vi "StopSplashScreen.vi"(8 "error in (no error)":errorcluster) -> (0 "error out":errorcluster)   [LabVIEW 2011]
uses:
  EnumFgvEventCommand.ctl
  ToSplashScreen.ctl
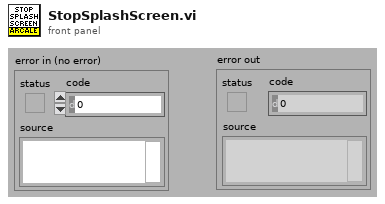
[diagram p1: front panel]
types:
  T1 = typedef "ToSplashScreen.ctl" = cluster{"Command":enum16{"Stop"}}
  T2 = typedef "EnumFgvEventCommand.ctl" = enum16{"Setup", "Cleanup", "Get"}
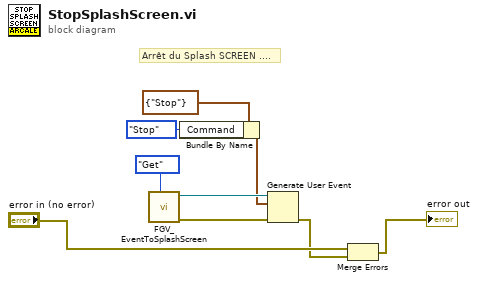
[diagram p0: block diagram]
diagram:
  # "Arrêt du Splash SCREEN ...."
  n1 = call "FGV_EventToSplashScreen.vi"("Command"=EnumFgvEventCommand."Get") -> ("error out"=w7:errorcluster, "ToSplashScreenEvent"=w8:refnum<user-event>)  [unwired: 9 in]
  n2 = Bundle By Name(cluster=T1 {"Command"=enum."Stop"} ("event data"), "Command"=enum16{"Stop"}."Stop") -> (w5:T1)
  n3 = Generate User Event(user event=w8, event data cluster=w5, error in=w7) -> (error out=w2:errorcluster)  [unwired: 1 out]
  n4 = Merge Errors("error in (no error)", w2) -> (→"error out":errorcluster)
